vi "TREE_Get First Parent Tag.vi"(8 "error in":errorcluster, 10 "tag in":string, 11 "Tree Ref":refnum<vi>) -> (0 "error out":errorcluster, 2 "tag out":string, 3 "Tree Ref":refnum<vi>)   [LabVIEW 2016]
doc: "Set a customize symbol for a item. Notice that all the symbol of items have the same symbol index will change. Set a new symbol index if you want to customize a single item."
panel:
  # "Input"
  # "Output"
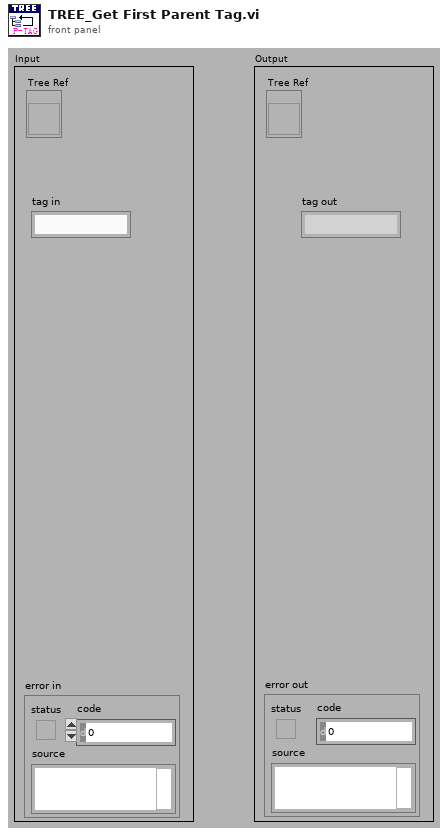
[diagram p1: front panel]
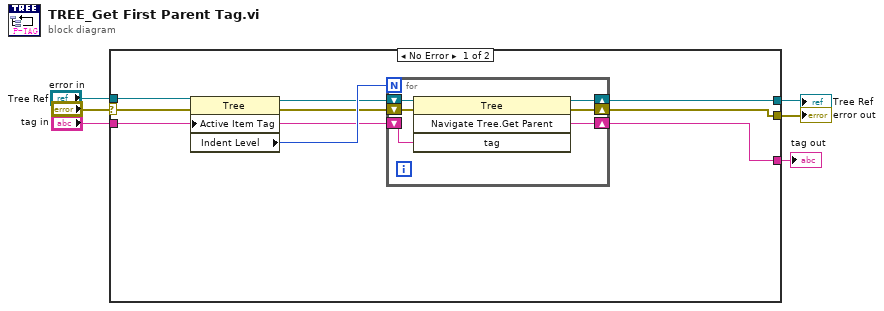
[diagram p0: block diagram]
diagram:
  n1 = case shown="No Error" "error in" {
    selector: "error in" -> [w12 w23]
    tunnel: [w10 w23] -> w6
    tunnel: [w8 w22] -> w4
    tunnel: "Tree Ref" -> [w13 w22]
    tunnel: "tag in" -> [w9 _]
    tunnel: [w7 _] -> w1
    frame No Error {
      n2 = property class="Tree"(reference=w13, error in=w12, "Active Item Tag"=w9) -> (reference out=w14:refnum<vi>, error out=w11:errorcluster, "Indent Level"=w15:i32)
      n3 = for {
        N: w15 -> [_]
        shift-right: [w19] -> w7
        shift-left: w9 -> [w21]
        shift-right: [w18] -> w8
        shift-left: w14 -> [w20]
        shift-right: [w16] -> w10
        shift-left: w11 -> [w17]
        n4 = invoke class="Tree" method="Navigate Tree.Get Parent"(reference=w20, error in=w17, "tag"=w21) -> (reference out=w18:refnum<vi>, error out=w16:errorcluster, "Navigate Tree:Get Parent"=w19:string)  [unwired: 1 in, 1 out]
      }
    }
    frame Error {
    }
  }
  "error out" <- w6
  "Tree Ref" <- w4
  "tag out" <- w1
